vi "Insert Bound View.vi"(8 "error in (no error)":errorcluster, 9 "Value Publication Time":timestamp, 10 "Selector Value":string, 11 "BoundViewManager in":refnum<class "BoundViewManager.lvclass">) -> (0 "error out":errorcluster, 3 "BoundViewManager out":refnum<class "BoundViewManager.lvclass">)   [LabVIEW 2020, in "MVA Framework.lvlib" / "BoundViewManager.lvlib" / "BoundViewManager.lvclass"]
doc: "插入绑定视图"
uses:
  BoundViewManager.lvclass
  <vilib>/ActorFramework/Message Enqueuer/Message Enqueuer.lvclass
  BoundViewManager.lvclass/BoundViewManager.ctl
  modules/composed-lookup-table/Source/LookupTable/LookupTable.lvclass/LookupTable.ctl
  modules/mva-viewable/Source/IViewable/IViewable Messages/Insert Front Panel Msg/Insert Front Panel Msg.lvclass/Insert Front Panel Msg.ctl
  <vilib>/ActorFramework/Message Enqueuer/Message Enqueuer.lvclass/Message Enqueuer.ctl
  5fa081a0-0653-487f-b15a-5ff6557eeb63.vi
  fd307117-ae16-4db7-ac68-5bdb8b1ee965.vi
  modules/composed-lookup-table/Source/LookupTable/Read Table Reference.vi
  5fa081a0-0653-487f-b15a-5ff6557eeb63.vi/5a7267ad-595e-4610-9ac2-8bef780848ff.vi
  <vilib>/ActorFramework/Message Enqueuer/Enqueue.vi
  fd307117-ae16-4db7-ac68-5bdb8b1ee965.vi/5a7267ad-595e-4610-9ac2-8bef780848ff.vi
  modules/mva-viewable/Source/IViewable/IViewable Messages/Insert Front Panel Msg/Insert Front Panel Msg.lvclass
  C:/Program Files/National Instruments/LabVIEW 2020/vi.lib/ActorFramework/Message/Message.lvclass
  <vilib>/ActorFramework/Message Priority Queue/Priority Enqueue.vi
  modules/composed-lookup-table/Source/LookupTable/LookupTable.lvclass
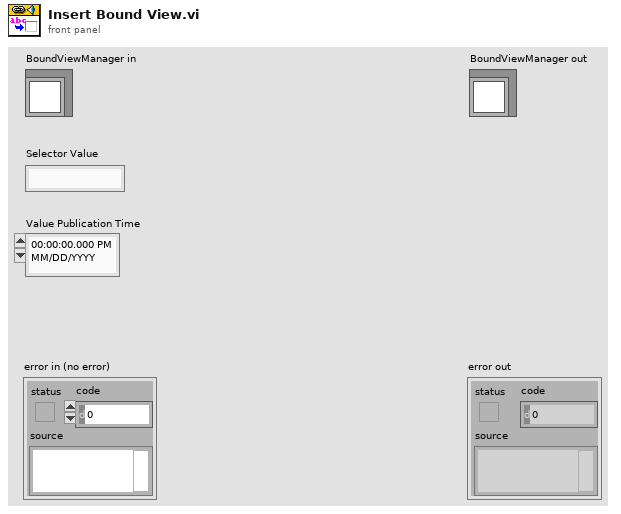
[diagram p1: front panel]
types:
  T1 = typedef "MVA Framework.lvlib/IViewable.lvlib/ProtectedSubpanel.lvclass/Protected Subpanel Reference.ctl" = refnum<data-value>
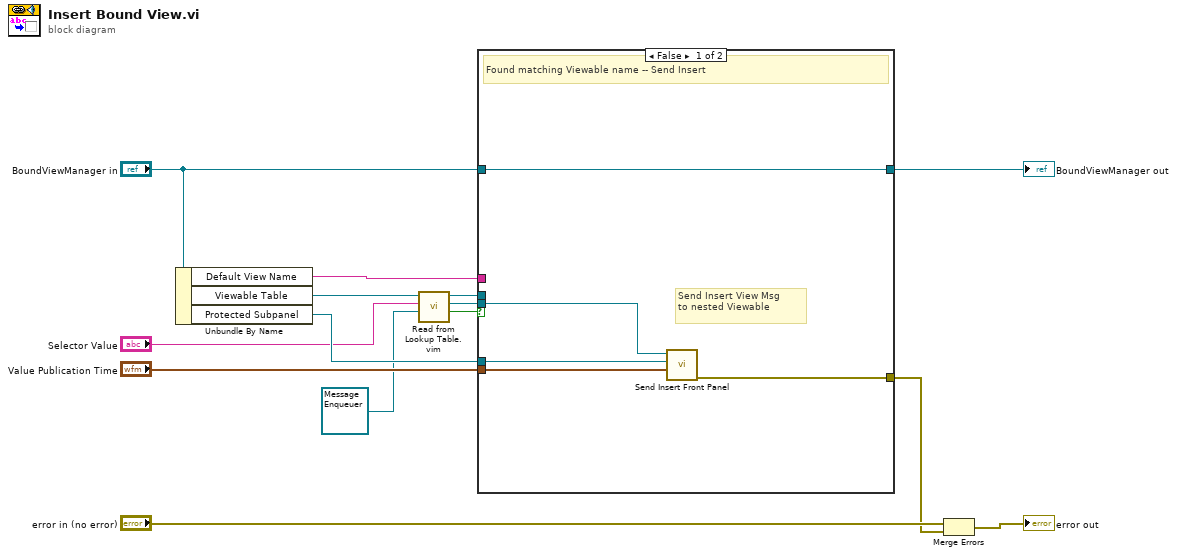
[diagram p0: block diagram]
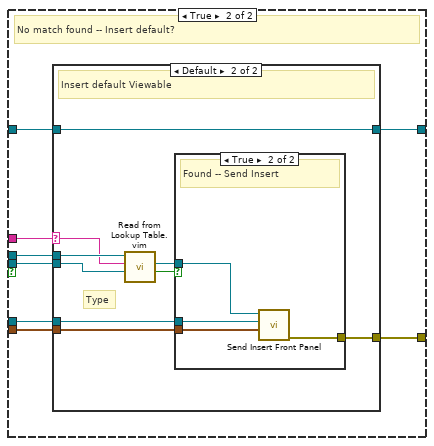
[diagram p2: hidden frame]
diagram:
  n1 = Unbundle By Name("BoundViewManager in") -> ("Default View Name"=w4:string, "Viewable Table"=w13:refnum<data-value>, "Protected Subpanel"=w12:T1)
  n2 = call "Read from Lookup Table.vim"("Type"=refnum<class "Message Enqueuer.lvclass"> refnum ("Message Enqueuer"), "Item Name"="Selector Value", "LookupTable Reference"=w13) -> ("Not Found?"=w9:bool, "Value"=w11:refnum<class "Message Enqueuer.lvclass">, "LookupTable Reference Out"=w2:refnum<data-value>)  [unwired: 5 in, 1 out]
  n3 = case shown="False" w9 {
    tunnel: w12 -> [w19 w24]
    tunnel: w11 -> [w15 w20]
    tunnel: "Value Publication Time" -> [w18 w23]
    tunnel: [w17 w22] -> w7
    tunnel: "BoundViewManager in" -> [w16 w27]
    tunnel: [w16 w26] -> w5
    tunnel: w4 -> [_ w25]
    tunnel: w2 -> [_ w21]
    frame False {
      # "Send Insert View Msg\nto nested Viewable"
      # "Found matching Viewable name -- Send Insert"
      n4 = call "Send Insert Front Panel.vi"("Request Time"=w18, "Protected Subpanel"=w19, "Message Enqueuer"=w15) -> ("error out"=w17:errorcluster)  [unwired: 7 in, 1 out]
    }
    frame True {
      # "No match found -- Insert default?"
      n5 = case shown="Default" w25 {
        selector: w25 -> [_ w32]
        tunnel: w27 -> [w28 w34]
        tunnel: [w28 w34] -> w26
        tunnel: w24 -> [_ w37]
        tunnel: w23 -> [_ w36]
        tunnel: [_ w35] -> w22
        tunnel: w21 -> [_ w33]
        tunnel: w20 -> [_ w29]
        frame "" {
          # "No default set -- No Viewable state change"
        }
        frame Default {
          # "Type"
          # "Insert default Viewable"
          n6 = call "Read from Lookup Table.vim"("Type"=w29, "Item Name"=w32, "LookupTable Reference"=w33) -> ("Not Found?"=w30:bool, "Value"=w31:refnum<class "Message Enqueuer.lvclass">)  [unwired: 5 in, 2 out]
          n7 = case shown="True" w30 {
            tunnel: w37 -> [_ w41]
            tunnel: w36 -> [_ w40]
            tunnel: [_ w39] -> w35
            tunnel: w31 -> [_ w38]
            frame False {
              # "Not found -- do nothing"
            }
            frame True {
              # "Found -- Send Insert"
              n8 = call "Send Insert Front Panel.vi"("Request Time"=w40, "Protected Subpanel"=w41, "Message Enqueuer"=w38) -> ("error out"=w39:errorcluster)  [unwired: 7 in, 1 out]
            }
          }
        }
      }
    }
  }
  "BoundViewManager out" <- w5
  n9 = Merge Errors("error in (no error)", w7) -> (→"error out":errorcluster)
